vi "getObjects.vi"(6 "type(ClassName)":string="Wire", 8 "error in (no error)":errorcluster, 11 "BlockDiagram in":refnum<class "BlockDiagram.lvclass">) -> (0 "error out":errorcluster, 2 "refs":refnum<vi>[](array[refnum]), 3 "BlockDiagram out":refnum<class "BlockDiagram.lvclass">)   [LabVIEW 2023, in "TLC_Scripto.lvlib" / "BlockDiagram.lvclass"]
uses:
  BlockDiagram.lvclass
  BlockDiagram.lvclass/BlockDiagram.ctl
  <vilib>/Utility/traverseref.llb/TRef TravTarget.ctl
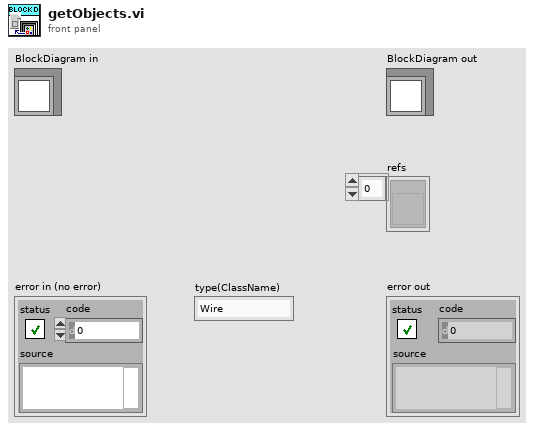
[diagram p1: front panel]
types:
  T1 = typedef "TRef TravTarget.ctl" = enum16{"FP", "BD", "Other"}
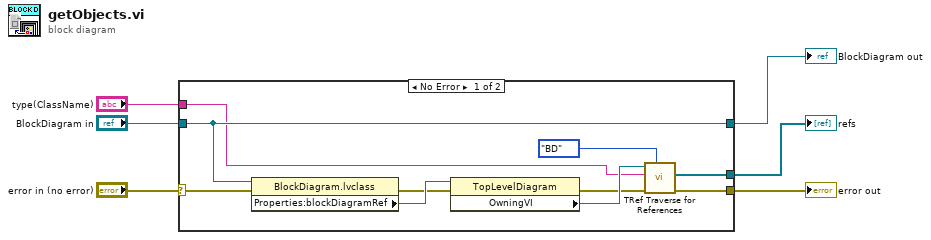
[diagram p0: block diagram]
diagram:
  n1 = case shown="No Error" "error in (no error)" {
    selector: "error in (no error)" -> [w10 w18]
    tunnel: [w8 w18] -> w5
    tunnel: [w13 w17] -> w3
    tunnel: "BlockDiagram in" -> [w13 w17]
    tunnel: "type(ClassName)" -> [w9 _]
    tunnel: [w7 _] -> w1
    frame No Error {
      n2 = property class="BlockDiagram.lvclass"(reference=w13, error in=w10) -> (error out=w11:errorcluster, "Properties:blockDiagramRef"=w12:refnum<vi>)  [unwired: 1 out]
      n3 = property on="Property Node" class="TopLevelDiagram"(reference=w12, error in=w11) -> (error out=w15:errorcluster, "OwningVI"=w16:refnum<vi>)  [unwired: 1 out]
      n4 = call <vilib>:"TRef Traverse for References.vi"("Traverse Target"=TRef_TravTarget."BD", "error in (no error)"=w15, "Class Name"=w9, "VI Refnum"=w16) -> ("error out"=w8:errorcluster, "References"=w7:refnum<vi>[])  [unwired: 1 in, 5 out]
    }
    frame Error {
    }
  }
  "error out" <- w5
  "BlockDiagram out" <- w3
  "refs" <- w1
